vi "Configure Fully Custom Loops.vi"(8 "error in (no error)":errorcluster, 10 "FullyCustom Configs":T1[](array[typedef]), 11 "FPGA Interface Base in":refnum<class "FPGA Interface Base.lvclass">) -> (0 "error out":errorcluster, 3 "FPGA Interface Base out":refnum<class "FPGA Interface Base.lvclass">)   [LabVIEW 2011, in "Engine Sim RT.lvlib"]
uses:
  Engine Sim RT.lvlib
  <userlib>/_FPGA Interface Advanced Tools/FPGA Interface Base/FPGA Interface Base.lvclass
  Shared/FullyCustomConfig.ctl
  Shared/FullyCustomProfileConfig.ctl
  Shared/FullyCustomCommMode.ctl
  <userlib>/_FPGA Interface Advanced Tools/FPGA Interface Base/FPGA Write By Name - U8.vi
  <userlib>/_FPGA Interface Advanced Tools/FPGA Interface Base/FPGA Write By Name - Boolean.vi
  <userlib>/_FPGA Interface Advanced Tools/FPGA Interface Base/FPGA Write FIFO By Name - U64.vi
  <userlib>/_FPGA Interface Advanced Tools/FPGA Interface Base/FPGA Write By Name - U64.vi
  Engine Simulation Shared.lvlib
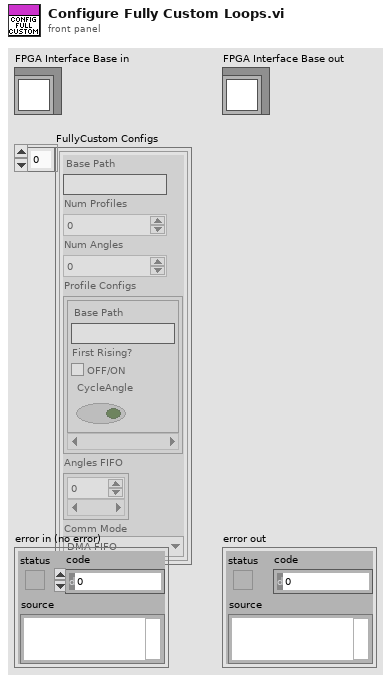
[diagram p1: front panel]
types:
  T1 = typedef "Engine Simulation Shared.lvlib/FullyCustomConfig.ctl" = cluster{"Base Path":string, "Num Profiles":u8, "Num Angles":u8, "Profile Configs":T2[], "Angles FIFO":u64[], "Comm Mode":T3}
  T2 = typedef "Engine Simulation Shared.lvlib/FullyCustomProfileConfig.ctl" = cluster{"Base Path":string, "First Rising?":bool, "CycleAngle":bool}
  T3 = typedef "Engine Simulation Shared.lvlib/FullyCustomCommMode.ctl" = enum16{"DMA FIFO", "FP Data Transfer"}
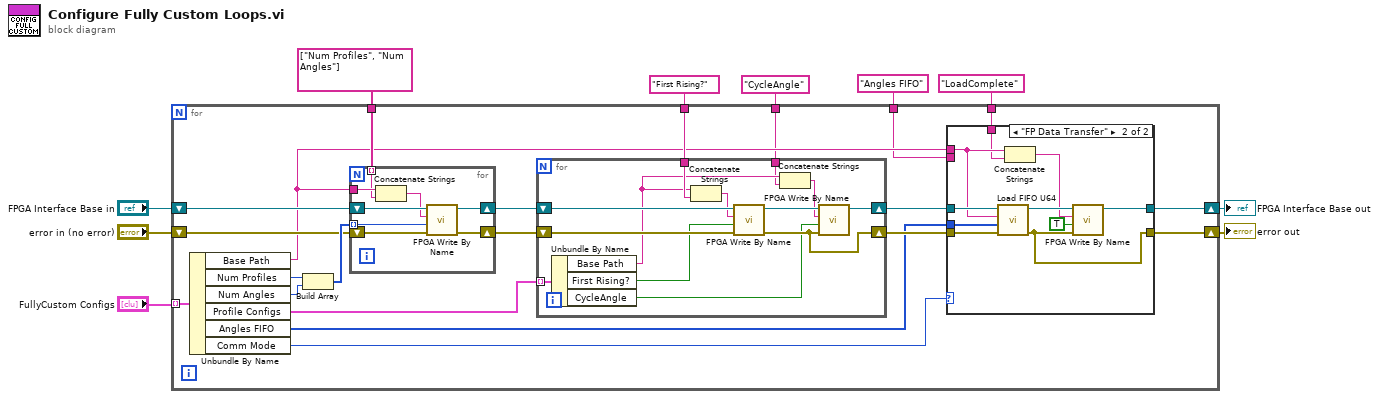
[diagram p0: block diagram]
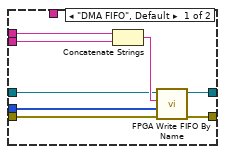
[diagram p2: hidden frame]
diagram:
  n1 = for {
    shift-right: [w18] -> w10
    shift-left: "FPGA Interface Base in" -> [w26]
    shift-right: [w17] -> w8
    shift-left: "error in (no error)" -> [w25]
    tunnel: "FullyCustom Configs" -> [w31] mode=indexing
    tunnel: string[] ["Num Profiles", "Num Angles"] -> [w27]
    tunnel: "First Rising?" ("Base Path") -> [w21]
    tunnel: "Angles FIFO" ("Base Path") -> [w13]
    tunnel: "LoadComplete" ("Base Path") -> [w14]
    tunnel: "CycleAngle" ("Base Path") -> [w11]
    n2 = Unbundle By Name(w31) -> ("Base Path"=w15:string, "Num Profiles"=w30:u8, "Num Angles"=w29:u8, "Profile Configs"=w22:T2[], "Angles FIFO"=w16:u64[], "Comm Mode"=w12:T3)
    n3 = Build Array(w30, w29) -> (w28:u8[])
    n4 = for {
      tunnel: w28 -> [w69] mode=indexing
      shift-right: [w63] -> w23
      shift-left: w25 -> [w70]
      shift-right: [w67] -> w24
      shift-left: w26 -> [w68]
      tunnel: w15 -> [w66]
      tunnel: w27 -> [w65] mode=indexing
      n5 = Concatenate Strings(w66, w65) -> (w64:string)
      n6 = call-poly <userlib>:"FPGA Write By Name.vi"("error in (no error)"=w70, "Value"=w69, "Control"=w64, "FPGA Session In"=w68) -> ("error out"=w63:errorcluster, "FPGA Session Out"=w67:refnum<class "FPGA Interface Base.lvclass">)  [unwired: 6 in]
    }
    n7 = for {
      tunnel: w22 -> [w59] mode=indexing
      shift-right: [w55] -> w20
      shift-left: w23 -> [w62]
      shift-right: [w56] -> w19
      shift-left: w24 -> [w61]
      tunnel: w21 -> [w58]
      tunnel: w11 -> [w53]
      n8 = Unbundle By Name(w59) -> ("Base Path"=w54:string, "First Rising?"=w51:bool, "CycleAngle"=w50:bool)
      n9 = Concatenate Strings(w54, w58) -> (w60:string)
      n10 = call-poly <userlib>:"FPGA Write By Name.vi"("error in (no error)"=w62, "Value"=w51, "Control"=w60, "FPGA Session In"=w61) -> ("error out"=w55:errorcluster, "FPGA Session Out"=w57:refnum<class "FPGA Interface Base.lvclass">)  [unwired: 6 in]
      n11 = Concatenate Strings(w54, w53) -> (w52:string)
      n12 = call-poly <userlib>:"FPGA Write By Name.vi"("error in (no error)"=w55, "Value"=w50, "Control"=w52, "FPGA Session In"=w57) -> ("FPGA Session Out"=w56:refnum<class "FPGA Interface Base.lvclass">)  [unwired: 6 in, 1 out]
    }
    n13 = case shown="\"FP Data Transfer\"" w12 {
      tunnel: w20 -> [w34 w49]
      tunnel: w19 -> [w36 w48]
      tunnel: [w32 w47] -> w18
      tunnel: [w33 w40] -> w17
      tunnel: w16 -> [w35 w46]
      tunnel: w15 -> [w38 w45]
      tunnel: w14 -> [_ w44]
      tunnel: w13 -> [w37 _]
      frame "DMA FIFO", Default {
        n14 = Concatenate Strings(w38, w37) -> (w39:string)
        n15 = call-poly <userlib>:"FPGA Write FIFO By Name.vi"("error in (no error)"=w34, "Data"=w35, "FIFO"=w39, "FPGA Session In"=w36) -> ("error out"=w33:errorcluster, "FPGA Session Out"=w32:refnum<class "FPGA Interface Base.lvclass">)  [unwired: 5 in, 1 out]
      }
      frame "FP Data Transfer" {
        n16 = call "Load FIFO U64.vi"("error in (no error)"=w49, "Data"=w46, "Base Path"=w45, "FPGA Session In"=w48) -> ("error out"=w40:errorcluster, "FPGA Session Out"=w42:refnum<class "FPGA Interface Base.lvclass">)  [unwired: 6 in]
        n17 = Concatenate Strings(w45, w44) -> (w41:string)
        n18 = call-poly <userlib>:"FPGA Write By Name.vi"("error in (no error)"=w40, "Value"=TRUE, "Control"=w41, "FPGA Session In"=w42) -> ("FPGA Session Out"=w47:refnum<class "FPGA Interface Base.lvclass">)  [unwired: 6 in, 1 out]
      }
    }
  }
  "FPGA Interface Base out" <- w10
  "error out" <- w8
